vi "Calculate Mask Test Gate Query.vi"(8 "error in":errorcluster, 9 "Gate Type":i32(ring) items=["Time", "Points", "Frequency", "Cursors"], 10 "Calculation Channel":i32(ring) items=["Calc Channel 1", "Calc Channel 2", "Calc Channel 3", "Calc Channel 4"], 11 "Instrument Handle In":i32) -> (0 "error out":errorcluster, 1 "Stop":dbl, 2 "Start":dbl, 3 "Instrument Handle Out":i32)   [LabVIEW 8.6, in "ZTScopeM.lvlib"]
doc: "Query the mask test gate settings of the selected calculation channel."
uses:
  ZTScopeM.lvlib
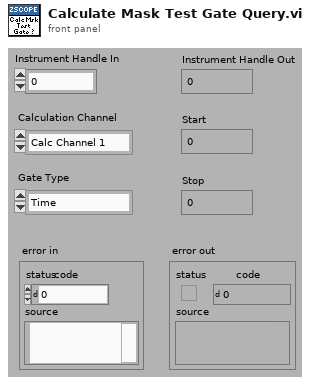
[diagram p1: front panel]
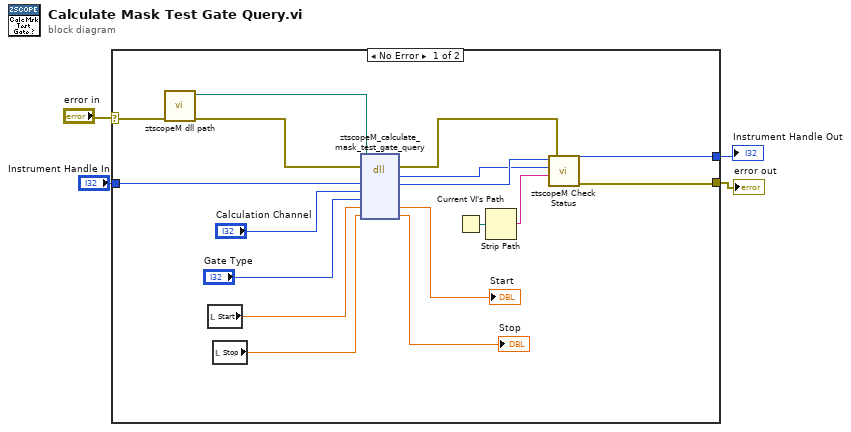
[diagram p0: block diagram]
diagram:
  n1 = case shown="No Error" "error in" {
    selector: "error in" -> [w8 w23]
    tunnel: [w15 w23] -> w2
    tunnel: "Instrument Handle In" -> [w21 w22]
    tunnel: [w14 w22] -> w1
    frame #0 {
      n2 = call "ztscopeM dll path.vi"("error in (no error)"=w8) -> ("error out"=w6:errorcluster, "<instrument>.dll path"=w7:path)  [unwired: 9 in]
      n3 = local read "Start"() -> (w11:dbl)
      n4 = local read "Stop"() -> (w9:dbl)
      n5 = dll-call lib="C:/Program Files (x86)/National Instruments/LabVIEW 2013/instr.lib/ztscopem/ztscopeM.dll" fn="ztscopeM_calculate_mask_test_gate_query"(path in=w7, error in=w6, "instrumentHandle"=w21, "calculationChannel"="Calculation Channel", "gate type"="Gate Type", "start"=w11, "stop"=w9) -> (error out=w5:errorcluster, w16:i32, "instrumentHandle"=w17:i32, "start"=→"Start":dbl, "stop"=→"Stop":dbl)  [unwired: 3 in, 1 out]
      n6 = Current VI's Path() -> (path=w19:path)
      n7 = Strip Path(path=w19) -> (name=w18:string)  [unwired: 1 out]
      n8 = call "ztscopeM Check Status.vi"("error in"=w5, "name of VI"=w18, "status (return code)"=w16, "instrument handle in"=w17) -> ("error out"=w15:errorcluster, "instrument handle out"=w14:i32)  [unwired: 2 in]
    }
    frame #1 {
    }
  }
  "Instrument Handle Out" <- w1
  "error out" <- w2
